vi "Set_PS2_18V.vi"(3 "error in":errorcluster) -> (10 "error out":errorcluster)   [LabVIEW 2015]
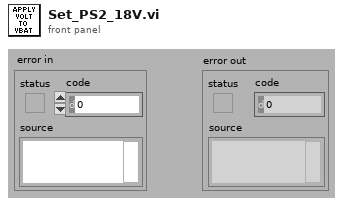
[diagram p1: front panel]
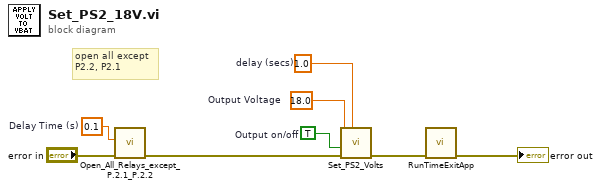
[diagram p0: block diagram]
diagram:
  w1 = 0.1  # Delay Time (s)
  w4 = TRUE  # Output on/off
  w5 = 1.0  # delay (secs)
  w6 = 18.0  # Output Voltage
  # "open all except \nP2.2, P2.1"
  n1 = call "Open_All_Relays_except_P.2.1_P.2.2.vi"("Delay Time (s)"=w1, "error in"="error in") -> ("error out"=w2:errorcluster)  [unwired: 8 in]
  n2 = call "Set_PS2_Volts.vi"("delay (secs)"=w5, "error in"=w2, "Output on/off"=w4, "Output Voltage"=w6) -> ("error out"=w7:errorcluster)  [unwired: 5 in, 2 out]
  n3 = call "RunTimeExitApp.vi"("error in (no error)"=w7) -> ("error out"=→"error out":errorcluster)  [unwired: 10 in]
